vi "PRIOR_IFilterPositionSet.vi"(8 "error in (no error)":errorcluster, 9 "Position":i16=1 min=1 max=10 step=1, 10 "Wheel":i32=1, 11 "PRIORLib In":T1) -> (0 "error out":errorcluster, 3 "PRIORLib Out":T1)   [LabVIEW 2010]
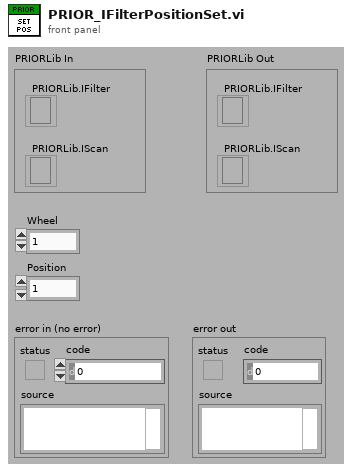
[diagram p1: front panel]
types:
  T1 = cluster{"PRIORLib.IFilter":refnum<k7>, "PRIORLib.IScan":refnum<k7>}
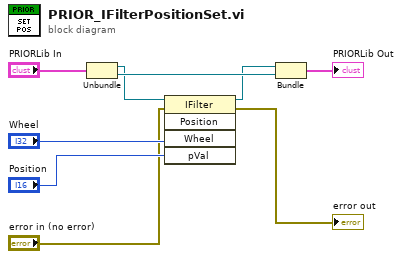
[diagram p0: block diagram]
diagram:
  n1 = Unbundle("PRIORLib In") -> ("PRIORLib.IFilter"=w2:refnum<k7>, "PRIORLib.IScan"=w4:refnum<k7>)
  n2 = invoke class="IFilter" method="Position"(reference=w2, error in="error in (no error)", "Wheel"="Wheel", "pVal"="Position") -> (reference out=w1:refnum<k7>, error out=→"error out":errorcluster)  [unwired: 1 in, 3 out]
  n3 = Bundle("PRIORLib.IFilter"=w1, "PRIORLib.IScan"=w4) -> (→"PRIORLib Out":T1)  [unwired: 1 in]
